vi "Convert Bitpacked Array.vi"(9 "Length":i32, 10 "Index":i32, 11 "Values":dbl[](array[numeric])) -> (3 "Numeric":u64)   [LabVIEW 2017, in "FPGA Addon Engine.lvlib"]
uses:
  FPGA Addon Engine.lvlib
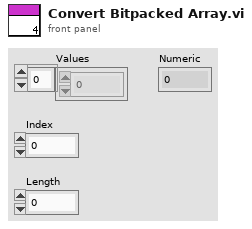
[diagram p1: front panel]
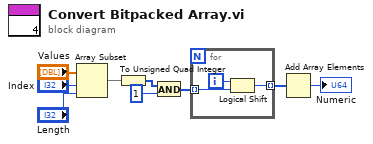
[diagram p0: block diagram]
diagram:
  n1 = Array Subset(array="Values", index="Index", length="Length") -> (w7:dbl[])
  n2 = To Unsigned Quad Integer(1:w7) -> (0:w6:u64[])
  n3 = And(x=w6, y=u64 1) -> (x .and. y?=w4:u64[])
  n4 = for {
    tunnel: w4 -> [w12] mode=indexing
    tunnel: [w10] -> w3 mode=indexing
    i -> [w11]
    n5 = Logical Shift(y=w11, x=w12) -> (x << y=w10:u64)
  }
  n6 = Add Array Elements(numeric array=w3) -> (sum=→"Numeric":u64)
